vi "Open.vi"(7 "I2C Channel (0)":u8, 8 "Error In":errorcluster, 9 "Resolution (dps)":enum16{"2000", "500", "250"}(ring), 10 "I2C Slave Address (0x69)":enum8{"0x68", "0x69"}(ring)=enum."0x69", 11 "LINX Resource":T1) -> (0 "Error Out":errorcluster, 1 "Resolution (dps)":enum16{"2000", "500", "250"}(ring), 3 "LINX Resource":T1)   [LabVIEW 2014, in "LMH-LINX.lvlib" / "PmodGYRO.lvlib"]
doc: "Open the specified I2C channel and initalize the PmodGYRO by powering it on and configuring it's resolution."
uses:
  <vilib>/MakerHub/LINX/Public/Sensors/Pmods/GYRO/PmodGYRO.lvlib
  <vilib>/MakerHub/LINX/LMH-LINX.lvlib
  <vilib>/MakerHub/LINX/Private/Type Defs/Platform.ctl
  <vilib>/MakerHub/LINX/Private/Type Defs/Interface.ctl
  <vilib>/MakerHub/LINX/Private/Device/Type Defs/TCP Config.ctl
  <vilib>/MakerHub/LINX/Private/Device/Device.lvlib
  <vilib>/MakerHub/LINX/Private/Device/Type Defs/Channels.ctl
  <vilib>/MakerHub/LINX/Private/Device/Type Defs/LINX Device Config.ctl
  <vilib>/MakerHub/LINX/Private/Type Defs/LINX Ref.ctl
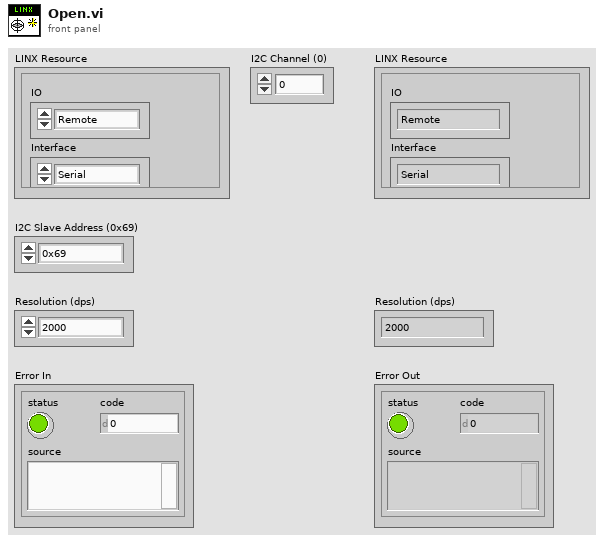
[diagram p1: front panel]
types:
  T1 = typedef "LMH-LINX.lvlib/LINX Ref.ctl" = cluster{"IO":T2, "Interface":T3, "LINX Device Config":T4}
  T2 = typedef "LMH-LINX.lvlib/Platform.ctl" = enum16{"Remote", "Local"}
  T3 = typedef "LMH-LINX.lvlib/Interface.ctl" = enum16{"Serial", "TCP"}
  T4 = typedef "LMH-LINX.lvlib/Device.lvlib/LINX Device Config.ctl" = cluster{"Interface":T3, "COM Port":refnum<visa-resource-name>, "TCP Configuration":T5, "Device Family":u8, "Device ID":u8, "Device Name":string, "TCP Ref":refnum<k5>, "Channels":T6}
  T5 = typedef "LMH-LINX.lvlib/Device.lvlib/TCP Config.ctl" = cluster{"IP Address":string, "Port":u16}
  T6 = typedef "LMH-LINX.lvlib/Channels.ctl" = cluster{"DI":u8[], "DO":u8[], "AI":u8[], "AO":u8[], "PWM":u8[], "QE":u8[], "UART":u8[], "I2C 2":u8[], "SPI":u8[], "CAN":u8[], "Servo":u8[], "AI Ref (V)":dbl, "AO Ref (V)":dbl, "AO Resolution (Bits)":u8}
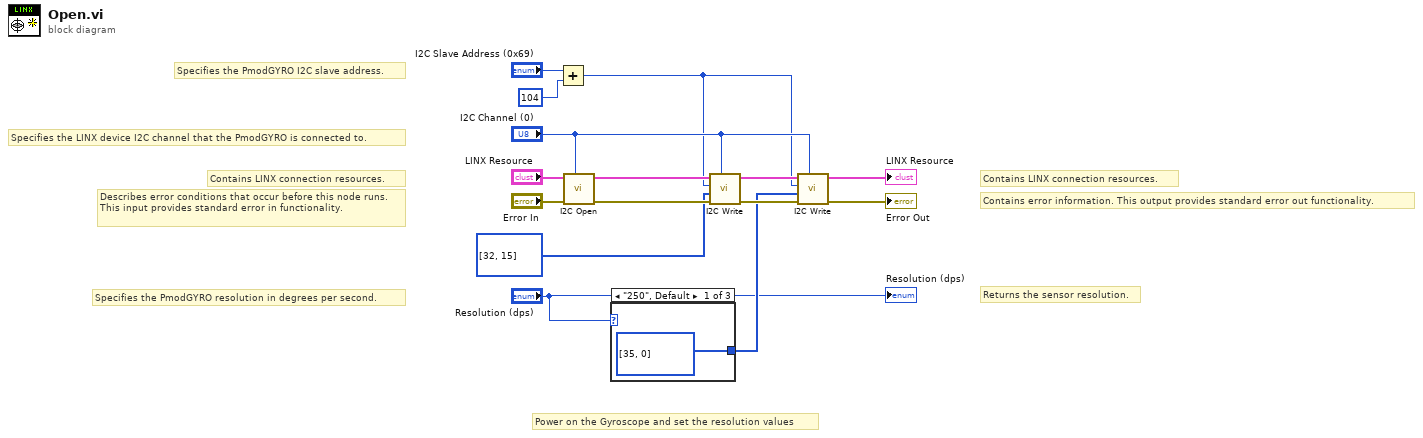
[diagram p0: block diagram]
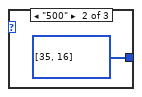
[diagram p2: hidden frame]
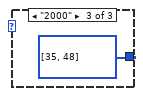
[diagram p3: hidden frame]
diagram:
  # "Specifies the PmodGYRO resolution in degrees per second."
  # "Specifies the PmodGYRO I2C slave address."
  # "Specifies the LINX device I2C channel that the PmodGYRO is connected to."
  # "Returns the sensor resolution."
  # "Contains LINX connection resources."
  # "Contains error information. This output provides standard error out functionality."
  # "Contains LINX connection resources."
  # "Describes error conditions that occur before this node runs. This input provides standard error in functionality."
  # "Power on the Gyroscope and set the resolution values"
  n1 = Add(x="I2C Slave Address (0x69)", y=u8 104) -> (x+y=w1:u8)
  n2 = call <vilib>:"I2C Open.vi"("I2C Channel (0)"="I2C Channel (0)", "Error In"="Error In", "LINX Resource"="LINX Resource") -> ("Error Out"=w10:errorcluster, "LINX Resource"=w9:T1)  [unwired: 7 in]
  n3 = case shown="\"250\", Default" "Resolution (dps)" {
    tunnel: [u8[] [35, 0] ("Data") u8[] [35, 16] ("Data") u8[] [35, 48] ("Data")] -> w8
    frame "250", Default {
    }
    frame "500" {
    }
    frame "2000" {
    }
  }
  n4 = call <vilib>:"I2C Write.vi"("I2C Channel"="I2C Channel (0)", "Error In"=w10, "Data"=u8[] [32, 15], "I2C Slave Address (0)"=w1, "LINX Resource"=w9) -> ("Error Out"=w11:errorcluster, "LINX Resource"=w14:T1)  [unwired: 5 in]
  n5 = call <vilib>:"I2C Write.vi"("I2C Channel"="I2C Channel (0)", "Error In"=w11, "Data"=w8, "I2C Slave Address (0)"=w1, "LINX Resource"=w14) -> ("Error Out"=→"Error Out":errorcluster, "LINX Resource"=→"LINX Resource":T1)  [unwired: 5 in]
  "Resolution (dps)" <- "Resolution (dps)"
